vi "Get Key Bool.vi"(7 "rel_path":string, 8 "error in (no error)":errorcluster, 9 "default value":bool, 10 "key":string, 11 "section":string) -> (0 "error out":errorcluster, 3 "value":bool)   [LabVIEW 2016]
uses:
  <vilib>/Utility/config.llb/Read Key (Boolean).vi
  <vilib>/Utility/config.llb/NI_LVConfig.lvlib
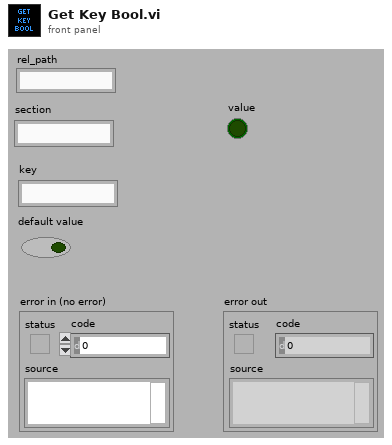
[diagram p1: front panel]
types:
  T1 = enum32{"invalid app kind", "Development System", "Run Time System", "Student Edition", "Embedded LabVIEW", "Evaluation", "Custom"}
  T2 = typedef "NI_LVConfig.lvlib/Config Data RefNum.ctl" = refnum<k1>
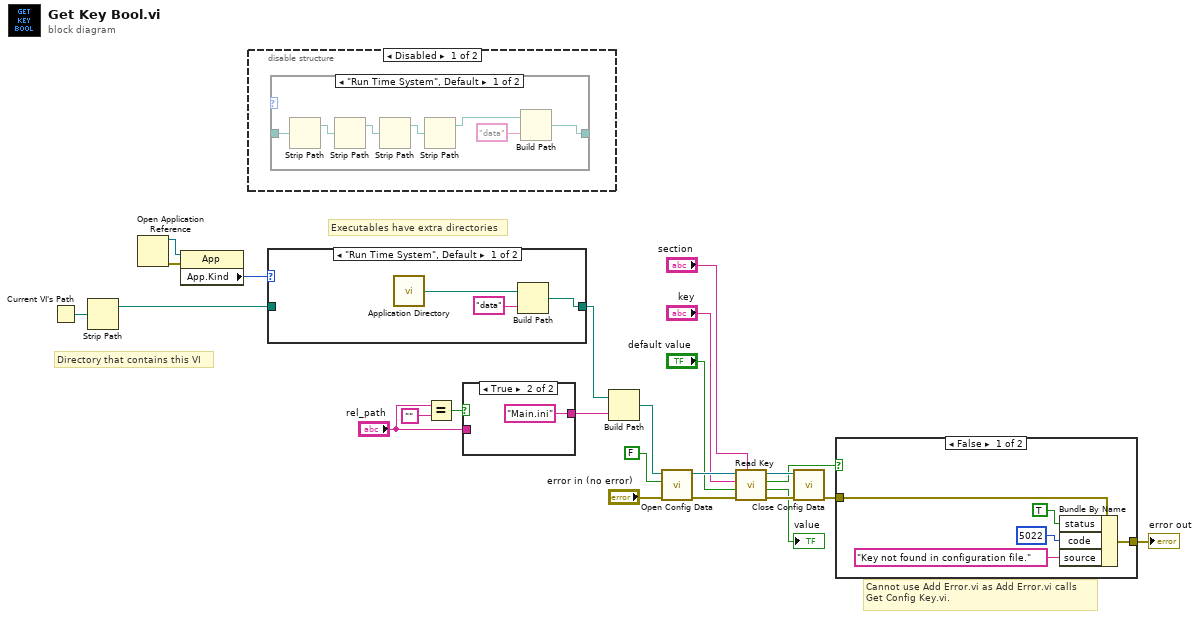
[diagram p0: block diagram]
diagram:
  # "Executables have extra directories"
  # "Cannot use Add Error.vi as Add Error.vi calls\nGet Config Key.vi."
  # "Directory that contains this VI"
  n1 = Current VI's Path() -> (path=w24:path)
  n2 = Strip Path(path=w24) -> (stripped path=w2:path)  [unwired: 1 out]
  n3 = Open Application Reference() -> (0:w4:errorcluster, 3:w5:refnum<vi>)  [unwired: 4 in]
  n4 = property class="App"(reference=w5, error in=w4) -> ("App.Kind"=w3:T1)  [unwired: 2 out]
  n5 = disable-structure shown="Disabled" {
    frame Disabled {
      n6 = case shown="\"Run Time System\", Default" {
        selector: _ -> [_ _]
        tunnel: _ -> [w25 w32]
        tunnel: [w30 w32] -> _
        frame "Run Time System", Default {
          n7 = Strip Path(path=w25) -> (stripped path=w27:path)  [unwired: 1 out]
          n8 = Strip Path(path=w27) -> (stripped path=w26:path)  [unwired: 1 out]
          n9 = Strip Path(path=w26) -> (stripped path=w31:path)  [unwired: 1 out]
          n10 = Strip Path(path=w31) -> (stripped path=w29:path)  [unwired: 1 out]
          n11 = Build Path(base path=w29, name or relative path="data") -> (appended path=w30:path)
        }
        frame "Development System" {
        }
      }
    }
    frame Enabled {
    }
  }
  n12 = case shown="\"Run Time System\", Default" w3 {
    tunnel: w2 -> [_ w36]
    tunnel: [w35 w36] -> w1
    frame "Run Time System", Default {
      n13 = call <vilib>:"Application Directory.vi"() -> ("Application Directory"=w33:path)
      n14 = Build Path(base path=w33, name or relative path="data") -> (appended path=w35:path)
    }
    frame "Development System" {
    }
  }
  n15 = Equal?(x="rel_path", y="") -> (x = y?=w11:bool)
  n16 = case shown="True" w11 {
    tunnel: [w37 "Main.ini" ("name or relative path")] -> w10
    tunnel: "rel_path" -> [w37 _]
    frame False {
    }
    frame True {
    }
  }
  n17 = Build Path(base path=w1, name or relative path=w10) -> (appended path=w23:path)
  n18 = call <vilib>:"Open Config Data.vi"("error in (no error)"="error in (no error)", "create file if necessary (T)"=FALSE, "configuration file path"=w23) -> ("error out"=w18:errorcluster, "refnum"=w21:T2)  [unwired: 6 in, 1 out]
  n19 = call-poly <vilib>:"Read Key.vi"("section"="section", "error in (no error)"=w18, "default value"="default value", "key"="key", "refnum"=w21) -> ("error out"=w16:errorcluster, "value"=→"value":bool, "found?"=w6:bool, "refnum out"=w15:T2)  [unwired: 3 in]
  n20 = call <vilib>:"Close Config Data.vi"("error in (no error)"=w16, "refnum"=w15) -> ("error out"=w7:errorcluster)  [unwired: 8 in, 1 out]
  n21 = case shown="False" w6 {
    tunnel: [w41 w44] -> w8
    tunnel: w7 -> [w39 w44]
    frame False {
      n22 = Bundle By Name(cluster=w39, "status"=TRUE, "code"=5022, "source"="Key not found in configuration file.") -> (w41:errorcluster)
    }
    frame True {
    }
  }
  "error out" <- w8
